vi "KE2260B Read Beeper Status.vi"(8 "error in (no error)":errorcluster, 11 "VISA resource name":refnum<visa-resource-name>) -> (0 "error out":errorcluster, 2 "Beeper Status":bool, 3 "VISA resource name out":refnum<visa-resource-name>)   [LabVIEW 2009, in "Keithley 2260B.lvlib"]
doc: "Returns the beeper status of the power supply."
uses:
  <instrlib>/Keithley 2260B/Keithley 2260B.lvlib
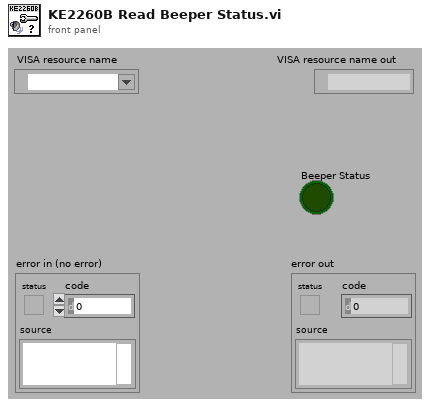
[diagram p1: front panel]
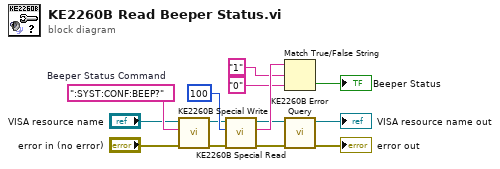
[diagram p0: block diagram]
diagram:
  w9 = ":SYST:CONF:BEEP?"  # Beeper Status Command
  n1 = call <instrlib>:"KE2260B Special Write.vi"("error in (no error)"="error in (no error)", "Write Buffer (\"\")"=w9, "VISA session"="VISA resource name") -> ("error out"=w11:errorcluster, "dup VISA session"=w10:refnum<visa-resource-name>)  [unwired: 6 in, 1 out]
  n2 = call <instrlib>:"KE2260B Special Read.vi"("error in (no error)"=w11, "byte count"=u32 100, "VISA session"=w10) -> ("error out"=w4:errorcluster, "read buffer"=w6:string, "dup VISA session"=w5:refnum<visa-resource-name>)  [unwired: 5 in, 1 out]
  n3 = Match True/False String(2:"0" ("false string"), 3:"1" ("true string"), 4:w6) -> (0:→"Beeper Status":bool)  [unwired: 1 out]
  n4 = call <instrlib>:"KE2260B Error Query.vi"("error in (no error)"=w4, "VISA resource name"=w5) -> ("error out"=→"error out":errorcluster, "VISA resource name out"=→"VISA resource name out":refnum<visa-resource-name>)  [unwired: 6 in, 2 out]
